vi "createQueryParameters.vi"(8 "error in (no error)":errorcluster, 10 "CoolerQuery":T1, 11 "CoolerSerialCommand in":refnum<class "CoolerSerialCommand.lvclass">) -> (0 "error out":errorcluster, 1 "commandName":string, 2 "commandId":string, 3 "CoolerSerialCommand out":refnum<class "CoolerSerialCommand.lvclass">, 4 "checkSum":string)   [LabVIEW 2016, in "CoolerSerialCommand.lvclass"]
uses:
  CoolerSerialCommand.lvclass
  typedefs/CoolerQuery.ctl
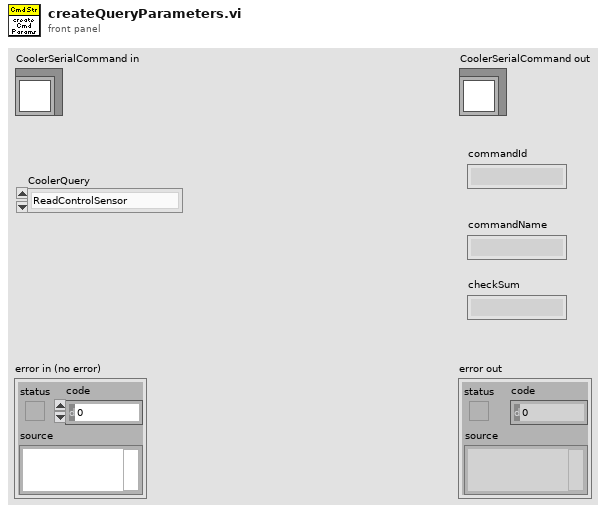
[diagram p1: front panel]
types:
  T1 = typedef "CoolerQuery.ctl" = enum16{"ReadControlSensor", "ReadSetTemperature", "ReadSupplyTemperature", "ReadExternalRTD", "ReadExternalThermistor", "ReadReturnTemperature", "ReadAmbientTemperature", "ReadProcessFlow", "ReadTECBank1Current", "ReadTECBank2Current", "ReadTEDriveLevel", "ReadAlarmStateLevel1", "ReadAlarmStateLevel21", "ReadAlarmStateLevel22", "ReadWarningStateLevel1", "ReadHighSupplyTempWarning", "ReadLowSupplyTempWarning", "ReadHighAmbientTempWarning", "ReadLowAmbientTempWarn ing", "ReadLowProcessFlowWarning", "ReadHighSupplyTempAlarm", "ReadLowSupplyTempAlarm", "ReadHighAmbientTempAlarm", "ReadLowAmbientTempAlarm", "ReadLowProcessFlowAlarm", "ReadPWMandRelayStatus", "ReadPIDStatus", "ReadUnitUpTime", "ReadFan1Speed", "ReadFan2Speed", "ReadFan3Speed", "ReadFan4Speed"}
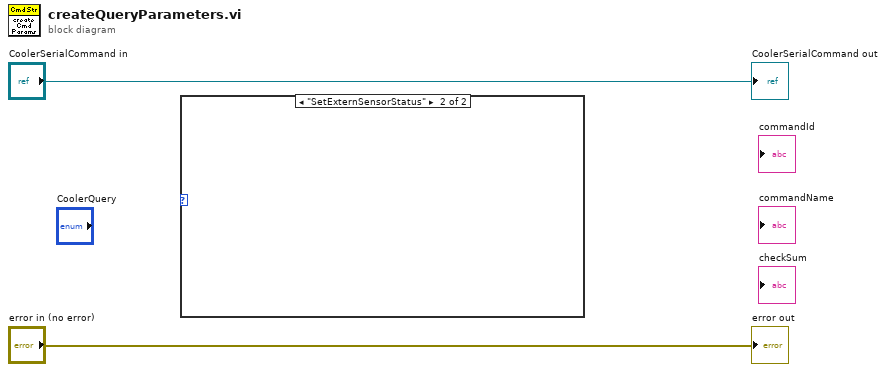
[diagram p0: block diagram]
diagram:
  n1 = case shown="\"SetExternSensorStatus\"" w1 {
    frame "None", Default {
    }
    frame "SetExternSensorStatus" {
    }
  }
  "error out" <- "error in (no error)"
  "CoolerSerialCommand out" <- "CoolerSerialCommand in"
